vi "Initialize Session.vi"(8 "error in (no error)":errorcluster, 11 "Python Toolkit in":refnum<class "Python Toolkit.lvclass">) -> (0 "error out":errorcluster, 3 "Python Toolkit out":refnum<class "Python Toolkit.lvclass">)   [LabVIEW 2018, in "Python Toolkit.lvclass"]
doc: "Initialize python session"
uses:
  Python Toolkit.lvclass
  Python Toolkit.lvclass/Python Toolkit.ctl
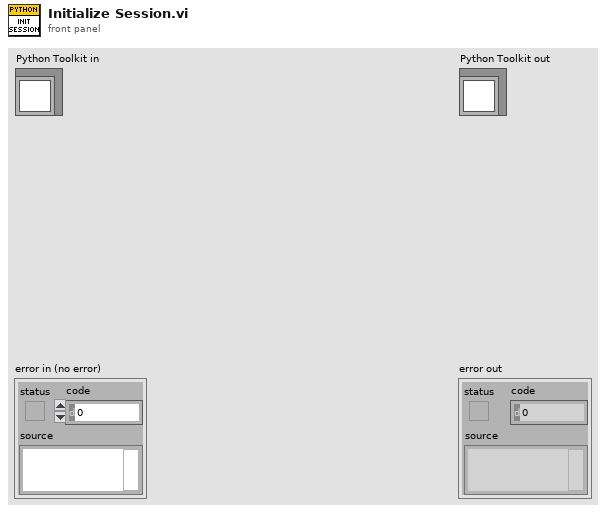
[diagram p1: front panel]
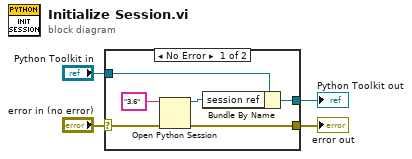
[diagram p0: block diagram]
diagram:
  n1 = case shown="No Error" "error in (no error)" {
    selector: "error in (no error)" -> [w7 w12]
    tunnel: [w6 w12] -> w3
    tunnel: [w9 w11] -> w1
    tunnel: "Python Toolkit in" -> [w10 w11]
    frame No Error {
      n2 = Open Python Session(python version="3.6" ("Python version"), 3:w7) -> (session out=w5:refnum<k35>, error out=w6:errorcluster)  [unwired: 1 in]
      n3 = Bundle By Name(cluster=w10, "session ref"=w5) -> (w9:refnum<class "Python Toolkit.lvclass">)
    }
    frame Error {
    }
  }
  "error out" <- w3
  "Python Toolkit out" <- w1
